vi "Update Report Previous RUNs.vi"(8 "error in (no error)":errorcluster, 10 "Previous RUN outcome":string, 11 "Monkey in":refnum<class "Monkey.lvclass">=refnum) -> (0 "error out":errorcluster, 3 "Monkey out":refnum<class "Monkey.lvclass">)   [LabVIEW 2020, in "CIRCUS_uServices.lvlib" / "Holy Trinity.lvlib" / "Monkey.lvlib" / "Monkey.lvclass"]
doc: "Add a timestamped line to the report message with the final result of the script"
uses:
  Monkey.lvclass
  TALOS/TALOS_PPL.lvlibp/Father of all uServices/Father of all uServices/Father of all uServices.lvclass
  TALOS/TALOS_PPL.lvlibp
  Run Utilities/Run Block/Run Block.lvclass
  C:/Users/marco/Documents/GitHub_Lab/CIRCUS/TALOS/TALOS_PPL.lvlibp/Ancestor/Ancestor/Ancestor.lvclass
  C:/Users/marco/Documents/GitHub_Lab/CIRCUS/TALOS/Actor Framework.lvlibp/1abvi3w/vi.lib/ActorFramework/Actor/Actor.lvclass
  C:/Users/marco/Documents/GitHub_Lab/CIRCUS/TALOS/TALOS_PPL.lvlibp/Father of all uServices/Father of all uServices/Father of all uServices.lvclass
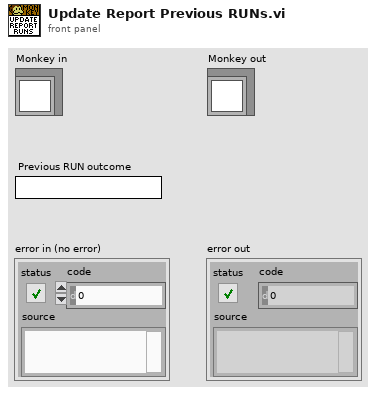
[diagram p1: front panel]
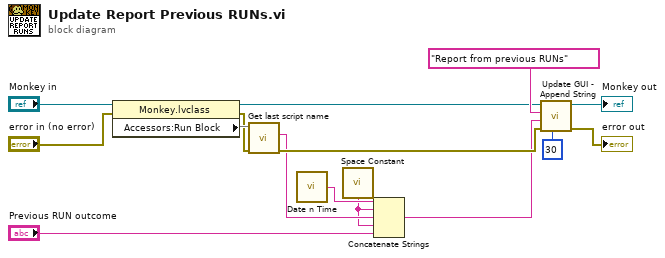
[diagram p0: block diagram]
diagram:
  n1 = property class="Monkey.lvclass"(reference="Monkey in", error in="error in (no error)") -> (reference out=w3:refnum<class "Monkey.lvclass">, error out=w4:errorcluster, "Accessors:Run Block"=w6)
  n2 = call-dynamic "Get last script name.vi"("error in (no error)"=w4, "Run Block in"=w6) -> ("error out"=w15:errorcluster, "Last script name"=w5:string)  [unwired: 7 in, 1 out]
  n3 = call "Date n Time.vi"() -> ("Date & Time"=w9:string)  [unwired: 5 in]
  n4 = call <vilib>:"Space Constant.vi"() -> ("String"=w2:string)
  n5 = Concatenate Strings(w9, w2, w5, w2, "Previous RUN outcome") -> (w10:string)
  n6 = call "Update GUI - Append String.vi"("Lines to keep"=u8 30, "error in (no error)"=w15, "String"=w10, "GUI Item Name"="Report from previous RUNs", "Father of all uServices in"=w3) -> ("error out"=→"error out":errorcluster, "Father of all uServices out"=→"Monkey out":refnum<class "Father of all uServices.lvclass">)  [unwired: 5 in]
